vi "XLP80_EA_Main.vi"(7 "Function":string, 8 "err in":errorcluster) -> (0 "err out":errorcluster)   [LabVIEW 2021]
uses:
  XLP80_Globals/Globals_Settings_XLP80.vi
  XLP80_EA_Globals.vi
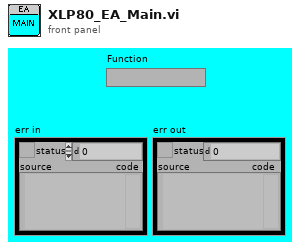
[diagram p1: front panel]
types:
  T1 = cluster{"Reku Simu":bool, "Stack Simu":bool, "Batterie Simu":bool}
  T2 = cluster{"Device Info Batterie":string[], "Device Info Stack":string[], "Device Info Rekuperation":string[]}
  T3 = cluster{"EA Batterie":errorcluster, "EA Stack":errorcluster, "EA Rekuperation":errorcluster}
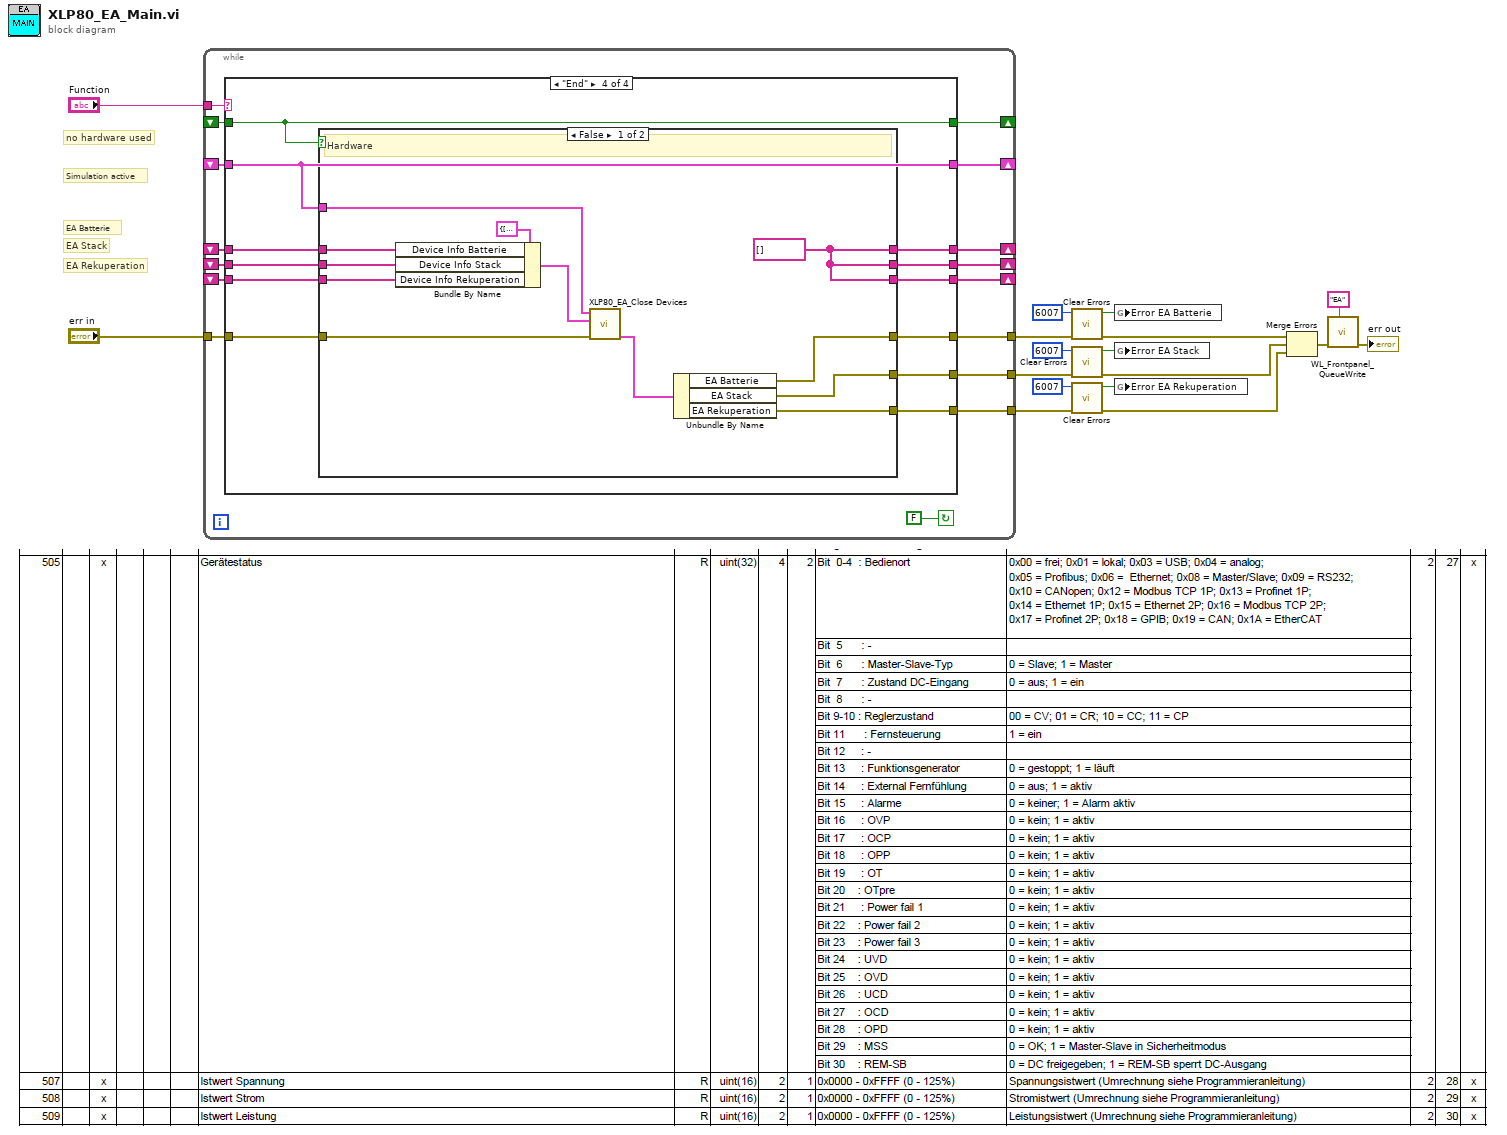
[diagram p0: block diagram]
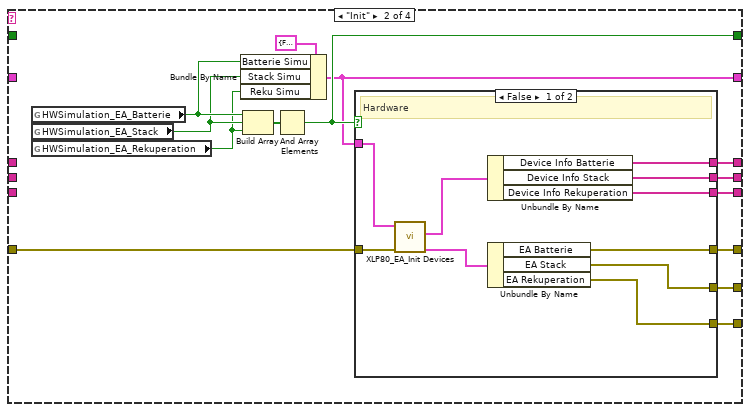
[diagram p3: hidden frame]
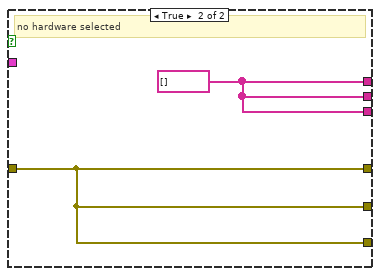
[diagram p4: hidden frame]
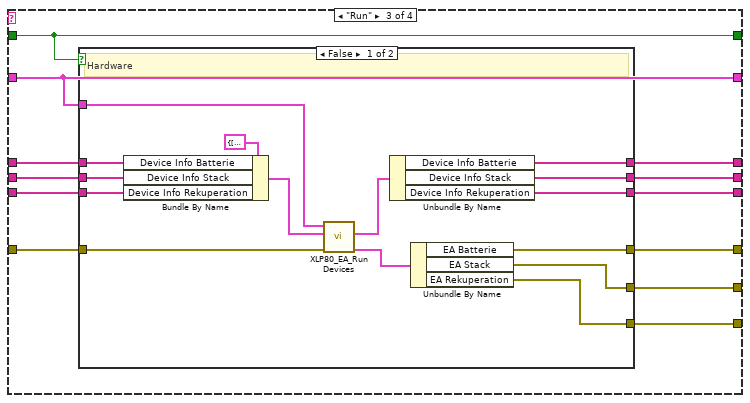
[diagram p5: hidden frame]
diagram:
  # "EA Rekuperation"
  # "EA Stack"
  # "EA Batterie"
  # "Simulation active"
  # "no hardware used"
  n1 = while {
    tunnel: "Function" -> [w32]
    shift-right: [w31] -> _
    shift-left: _ -> [w30]
    tunnel: "err in" -> [w29]
    tunnel: [w28] -> w15
    shift-right: [w27] -> _
    shift-left: _ -> [w26]
    shift-right: [w25] -> _
    shift-left: _ -> [w24]
    tunnel: [w23] -> w5
    tunnel: [w22] -> w4
    shift-right: [w21] -> _
    shift-left: _ -> [w20]
    shift-right: [w19] -> _
    shift-left: _ -> [w18]
    stop <- FALSE continue-if-true
    n2 = case shown="\"End\"" w32 {
      tunnel: [w39 w50 w75 w106] -> w31
      tunnel: w30 -> [w39 _ w75 w106]
      tunnel: w29 -> [w36 w53 w77 w108]
      tunnel: [w36 w52 w76 w107] -> w28
      tunnel: [w38 w51 w73 w104] -> w27
      tunnel: w26 -> [w38 _ w74 w105]
      tunnel: [w37 w47 w72 w103] -> w25
      tunnel: w24 -> [w37 _ w72 w103]
      tunnel: [w36 w46 w67 w102] -> w23
      tunnel: [w36 w45 w66 w101] -> w22
      tunnel: [w35 w44 w69 w98] -> w21
      tunnel: w20 -> [w35 _ w71 w100]
      tunnel: [w34 w43 w68 w97] -> w19
      tunnel: w18 -> [w34 _ w70 w99]
      frame Default {
      }
      frame "Init" {
        n3 = global read "Globals_Settings_XLP80.vi" "HWSimulation_EA_Batterie"() -> (w42:bool)
        n4 = global read "Globals_Settings_XLP80.vi" "HWSimulation_EA_Stack"() -> (w41:bool)
        n5 = global read "Globals_Settings_XLP80.vi" "HWSimulation_EA_Rekuperation"() -> (w40:bool)
        n6 = Bundle By Name(cluster=T1 {"Reku Simu"=FALSE, "Stack Simu"=FALSE, "Batterie Simu"=FALSE}, "Batterie Simu"=w42, "Stack Simu"=w41, "Reku Simu"=w40) -> (w47:T1)
        n7 = Build Array(w42, w41, w40) -> (w49:bool[])
        n8 = And Array Elements(Boolean array=w49) -> (logical AND=w50:bool)
        n9 = case shown="False" w50 {
          tunnel: w53 -> [w63 w64]
          tunnel: [w60 w64] -> w52
          tunnel: [w59 w65] -> w51
          tunnel: w47 -> [w62 _]
          tunnel: [w58 w64] -> w46
          tunnel: [w57 w64] -> w45
          tunnel: [w56 w65] -> w44
          tunnel: [w55 w65] -> w43
          frame False {
            # "Hardware"
            n10 = call "XLP80_EA_Init Devices.vi"("err in"=w63, "Simu EAs"=w62) -> ("Error EAs"=w61:T3, "Device Informations"=w54:T2)  [unwired: 8 in]
            n11 = Unbundle By Name(w54) -> ("Device Info Batterie"=w59:string[], "Device Info Stack"=w56:string[], "Device Info Rekuperation"=w55:string[])
            n12 = Unbundle By Name(w61) -> ("EA Batterie"=w60:errorcluster, "EA Stack"=w58:errorcluster, "EA Rekuperation"=w57:errorcluster)
          }
          frame True {
            w65 = string[] [] ("Device information out")
            # "no hardware selected"
          }
        }
      }
      frame "Run" {
        n13 = case shown="False" w75 {
          tunnel: w77 -> [w88 w93]
          tunnel: [w80 w93] -> w76
          tunnel: [w84 w96] -> w73
          tunnel: w74 -> [w91 w96]
          tunnel: w72 -> [w87 _]
          tunnel: w71 -> [w90 w95]
          tunnel: w70 -> [w89 w94]
          tunnel: [w83 w95] -> w69
          tunnel: [w82 w94] -> w68
          tunnel: [w79 w93] -> w67
          tunnel: [w78 w93] -> w66
          frame False {
            # "Hardware"
            n14 = Bundle By Name(cluster=T2 {"Device Info Batterie"=[], "Device Info Stack"=[], "Device Info Rekuperation"=[]} ("Device Informations"), "Device Info Batterie"=w91, "Device Info Stack"=w90, "Device Info Rekuperation"=w89) -> (w86:T2)
            n15 = call "XLP80_EA_Run Devices.vi"("err in"=w88, "Device Informations"=w86, "Simu EAs"=w87) -> ("Error EAs"=w81:T3, "Device Informations OUT"=w85:T2)  [unwired: 7 in]
            n16 = Unbundle By Name(w85) -> ("Device Info Batterie"=w84:string[], "Device Info Stack"=w83:string[], "Device Info Rekuperation"=w82:string[])
            n17 = Unbundle By Name(w81) -> ("EA Batterie"=w80:errorcluster, "EA Stack"=w79:errorcluster, "EA Rekuperation"=w78:errorcluster)
          }
          frame True {
            # "no hardware selected"
          }
        }
      }
      frame "End" {
        n18 = case shown="False" w106 {
          tunnel: w108 -> [w120 w123]
          tunnel: [w117 w123] -> w107
          tunnel: w105 -> [w112 w124]
          tunnel: [w109 w124] -> w104
          tunnel: w103 -> [w119 _]
          tunnel: [w116 w123] -> w102
          tunnel: [w115 w123] -> w101
          tunnel: w100 -> [w111 w122]
          tunnel: w99 -> [w110 w121]
          tunnel: [w109 w122] -> w98
          tunnel: [w109 w121] -> w97
          frame False {
            w109 = string[] [] ("Device information IN")
            # "Hardware"
            n19 = Bundle By Name(cluster=T2 {"Device Info Batterie"=[], "Device Info Stack"=[], "Device Info Rekuperation"=[]} ("Device Informations"), "Device Info Batterie"=w112, "Device Info Stack"=w111, "Device Info Rekuperation"=w110) -> (w113:T2)
            n20 = call "XLP80_EA_Close Devices.vi"("err in"=w120, "Device Informations"=w113, "Simu EAs"=w119) -> ("Error EAs"=w118:T3)  [unwired: 8 in]
            n21 = Unbundle By Name(w118) -> ("EA Batterie"=w117:errorcluster, "EA Stack"=w116:errorcluster, "EA Rekuperation"=w115:errorcluster)
          }
          frame True {
            # "no hardware selected"
          }
        }
      }
    }
  }
  n22 = call <vilib>:"Clear Errors.vi"("error in (no error)"=w15, "specific error code to clear (0: all)"=6007) -> ("error out"=w12:errorcluster, "specific error cleared?"=w13:bool)  [unwired: 4 in]
  n23 = call <vilib>:"Clear Errors.vi"("error in (no error)"=w5, "specific error code to clear (0: all)"=6007) -> ("error out"=w7:errorcluster, "specific error cleared?"=w11:bool)  [unwired: 4 in]
  n24 = call <vilib>:"Clear Errors.vi"("error in (no error)"=w4, "specific error code to clear (0: all)"=6007) -> ("error out"=w6:errorcluster, "specific error cleared?"=w8:bool)  [unwired: 4 in]
  n25 = global write "XLP80_EA_Globals.vi" "Error EA Batterie"(w13) -> ()
  n26 = global write "XLP80_EA_Globals.vi" "Error EA Stack"(w11) -> ()
  n27 = global write "XLP80_EA_Globals.vi" "Error EA Rekuperation"(w8) -> ()
  n28 = Merge Errors(w12, w7, w6) -> (w2:errorcluster)
  n29 = call "WL_Frontpanel_QueueWrite.vi"("Command (error only)"="EA", "err in"=w2) -> ("err out"=→"err out":errorcluster)  [unwired: 9 in]
